vi "json Parse U32 Array - string path.vi"(8 "error in (no error)":errorcluster, 9 "default":u32[](array[numeric]), 10 "path":string, 11 "JSON Document in":refnum<class "JSON Document.lvclass">) -> (0 "error out":errorcluster, 1 "defaulted?":bool, 2 "value":u32[](array[numeric]), 3 "JSON Document out":refnum<class "JSON Document.lvclass">, 4 "elements defaulted?":bool[](array[boolean]))   [LabVIEW 2015, in "JSON Document.lvclass"]
uses:
  JSON Document.lvclass
  json Parse U32 - string path.vi
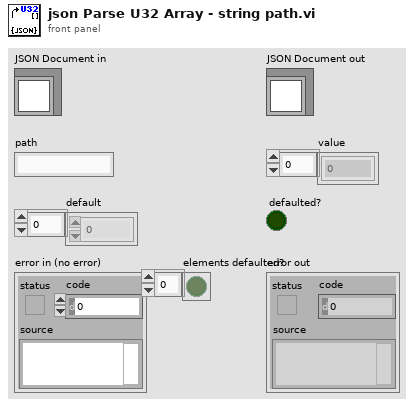
[diagram p1: front panel]
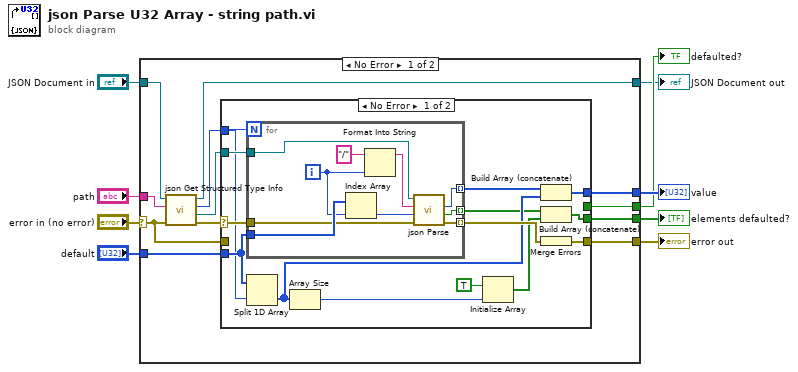
[diagram p0: block diagram]
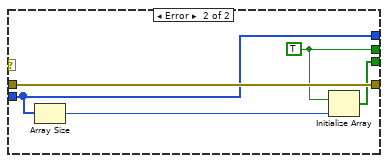
[diagram p2: hidden frame]
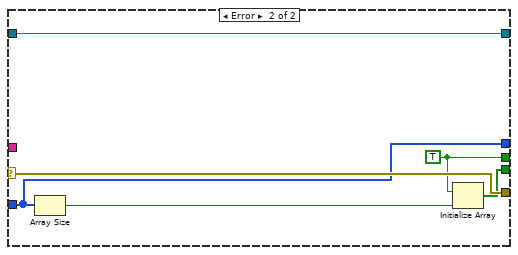
[diagram p3: hidden frame]
diagram:
  n1 = case shown="No Error" "error in (no error)" {
    selector: "error in (no error)" -> [w21 w56]
    tunnel: [w20 w56] -> w1
    tunnel: [w12 w55] -> w2
    tunnel: "JSON Document in" -> [w13 w55]
    tunnel: "default" -> [w18 w54]
    tunnel: "path" -> [w11 _]
    tunnel: [w19 w54] -> w5
    tunnel: [w17 w52] -> w3
    tunnel: [w10 w51] -> w4
    frame No Error {
      n2 = call "json Get Structured Type Info.vi"("error in (no error)"=w21, "path"=w11, "JSON Document in"=w13) -> ("error out"=w15:errorcluster, "value out"=w14:refnum<class "JSON Document.lvclass">, "count"=w16:i32, "JSON Document out"=w12:refnum<class "JSON Document.lvclass">)  [unwired: 5 in]
      n3 = case shown="No Error" w15 {
        selector: w15 -> [w35 _]
        tunnel: [w29 w49] -> w19
        tunnel: w16 -> [w22 _]
        tunnel: w18 -> [w31 w49]
        tunnel: [w33 w50] -> w20
        tunnel: w21 -> [_ w50]
        tunnel: w14 -> [w32 _]
        tunnel: [_ w47] -> w17
        tunnel: [w23 w46] -> w10
        frame No Error {
          n4 = for {
            N: w22 -> [_]
            tunnel: [w39] -> w34 mode=indexing
            tunnel: [w38] -> w30 mode=indexing
            tunnel: w31 -> [w44]
            tunnel: w35 -> [w40]
            tunnel: w32 -> [w43]
            tunnel: [w36] -> w25 mode=indexing
            i -> [w37]
            n5 = Index Array(array=w44, index=w37) -> (element=w41:u32)
            n6 = Format Into String(initial string="/", w37) -> (resulting string=w42:string)  [unwired: 2 in, 1 out]
            n7 = call-poly "json Parse.vi"("error in (no error)"=w40, "default"=w41, "path"=w42, "JSON Document in"=w43) -> ("error out"=w39:errorcluster, "defaulted?"=w36:bool, "value"=w38:u32)  [unwired: 4 in, 1 out]
          }
          n8 = Split 1D Array(array=w31, index=w22) -> (second subarray=w28:u32[])  [unwired: 1 out]
          n9 = Array Size(array=w28) -> (size(s)=w27:i32)
          n10 = Initialize Array(TRUE ("found?"), w27) -> (w24:bool[])
          n11 = Build Array (concatenate)(w30, w28) -> (w29:u32[])
          n12 = Build Array (concatenate)(w25, w24) -> (w23:bool[])
          n13 = Merge Errors(w34) -> (w33:errorcluster)
        }
        frame Error {
          w47 = TRUE ("found?")
          n14 = Array Size(array=w49) -> (size(s)=w48:i32)
          n15 = Initialize Array(w47, w48) -> (w46:bool[])
        }
      }
    }
    frame Error {
      w52 = TRUE ("found?")
      n16 = Array Size(array=w54) -> (size(s)=w53:i32)
      n17 = Initialize Array(w52, w53) -> (w51:bool[])
    }
  }
  "error out" <- w1
  "JSON Document out" <- w2
  "value" <- w5
  "defaulted?" <- w3
  "elements defaulted?" <- w4
